vi "LoadModel.vi"(8 "error in (no error)":errorcluster, 11 "View in":refnum<class "View.lvclass">) -> (0 "error out":errorcluster, 3 "View out":refnum<class "View.lvclass">)   [LabVIEW 2020, in "Page2.lvlib" / "View.lvclass"]
uses:
  View.lvclass
  View.lvclass/View.ctl
  Controller/Controller.lvclass
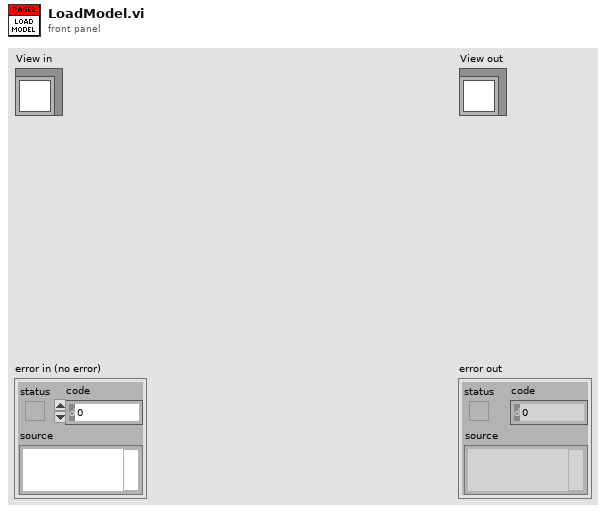
[diagram p1: front panel]
types:
  T1 = cluster{"Setting":refnum<vi>, "Time (s)":refnum<vi>, "Main Test Folder":refnum<vi>}
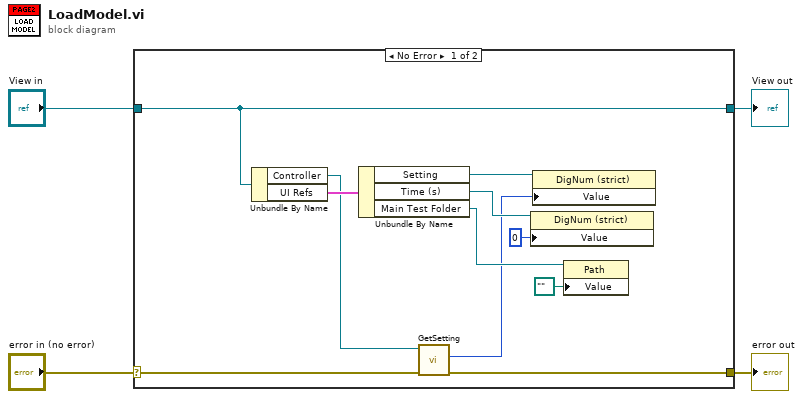
[diagram p0: block diagram]
diagram:
  n1 = case shown="No Error" "error in (no error)" {
    selector: "error in (no error)" -> [w7 w17]
    tunnel: [w8 w17] -> w3
    tunnel: [w15 w16] -> w1
    tunnel: "View in" -> [w15 w16]
    frame No Error {
      n2 = Unbundle By Name(w15) -> ("Controller"=w6:refnum<class "Controller.lvclass">, "UI Refs"=w14:T1)
      n3 = Unbundle By Name(w14) -> ("Setting"=w13:refnum<vi>, "Time (s)"=w12:refnum<vi>, "Main Test Folder"=w11:refnum<vi>)
      n4 = call "GetSetting.vi"("error in (no error)"=w7, "Controller in"=w6) -> ("error out"=w8:errorcluster, "Setting"=w9:u32)  [unwired: 7 in, 1 out]
      n5 = property class="DigNum (strict)"(reference=w12, "Value"=u32 0) -> ()  [unwired: 1 in, 2 out]
      n6 = property class="DigNum (strict)"(reference=w13, "Value"=w9) -> ()  [unwired: 1 in, 2 out]
      n7 = property class="Path"(reference=w11, "Value"=path "") -> ()  [unwired: 1 in, 2 out]
    }
    frame Error {
    }
  }
  "error out" <- w3
  "View out" <- w1
